vi "Example Import.vi"() -> ()   [LabVIEW 2019]
doc: "Example VI to import a VI Snippet (*.png) programmatically into a new VI.\n\nCreated by: Ryan Pacini"
uses:
  VI Snippet.lvlib
panel:
  in  "Copy to (\"VI\")":enum8{"VI", "Clipboard"}(ring)
  in  "VI Snippet (*.png)":path=path "C:/Projects/git/labview_snippet/src/Images/example.png"
  out "Preview":picture
  out "error out":errorcluster
  # "Import a VI Snippet (*.png) programmatically"
  # "(See Block Diagram for Instructions)"
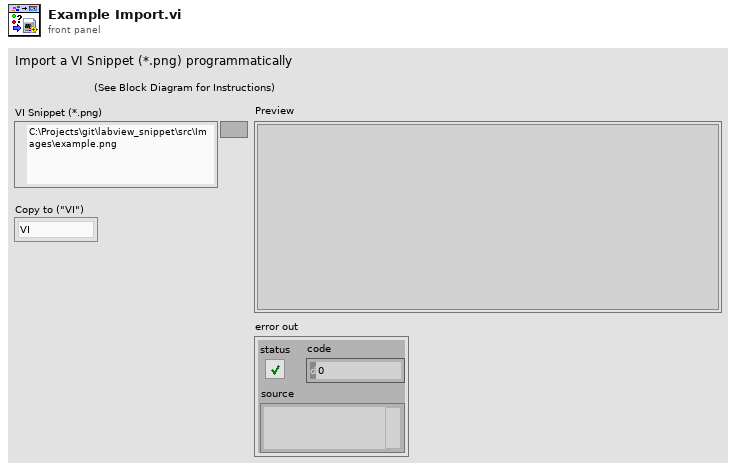
[diagram p1: front panel]
types:
  T1 = typedef "imagedata.ctl" = cluster{"image type":i32, "image depth":i32, "image":u8[], "mask":u8[], "colors":u32[], "Rectangle":cluster{"left":i16, "top":i16, "right":i16, "bottom":i16}}
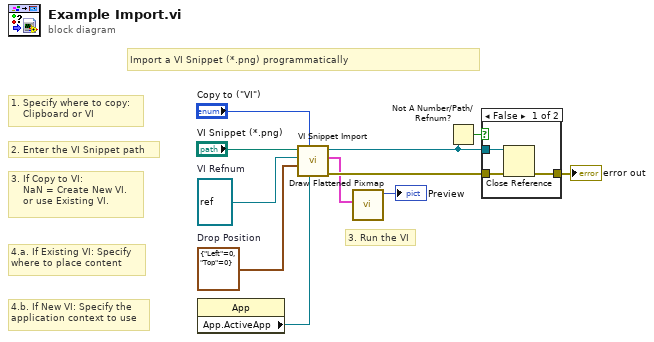
[diagram p0: block diagram]
diagram:
  w1 = cluster{"Left":i32, "Top":i32} {"Left"=0, "Top"=0}  # Drop Position
  w2 = refnum<vi> refnum  # VI Refnum
  # "4.a. If Existing VI: Specify\nwhere to place content"
  # "3. If Copy to VI:\n    NaN = Create New VI.\n    or use Existing VI."
  # "4.b. If New VI: Specify the\napplication context to use"
  # "1. Specify where to copy:\n    Clipboard or VI"
  # "3. Run the VI"
  # "2. Enter the VI Snippet path"
  # "Import a VI Snippet (*.png) programmatically"
  n1 = property class="App"() -> ("App.ActiveApp"=w3:refnum<vi>)  [unwired: 2 in, 2 out]
  n2 = call "VI Snippet Import.vi"("App Refnum (New VI only)"=w3, "Copy to (\"VI\")"="Copy to (\"VI\")", "Drop Position (0, 0)"=w1, "VI Refnum in (NaN=New VI)"=w2, "VI Snippet Path (*.png)"="VI Snippet (*.png)") -> ("error out"=w11:errorcluster, "Image Data out"=w8:T1, "VI Refnum out"=w5:refnum<vi>)  [unwired: 3 in, 1 out]
  n3 = call <vilib>:"Draw Flattened Pixmap.vi"("image data"=w8) -> ("new picture"=→"Preview":picture)  [unwired: 8 in]
  n4 = Not A Number/Path/Refnum?(number/path/refnum=w5) -> (NaN/Path/Refnum?=w4:bool)
  n5 = case shown="False" w4 {
    tunnel: w11 -> [w14 w15]
    tunnel: [w13 w15] -> w10
    tunnel: w5 -> [w12 _]
    frame False {
      n6 = Close Reference(reference=w12, error in (no error)=w14) -> (error out=w13:errorcluster)
    }
    frame True {
    }
  }
  "error out" <- w10
